vi "ThresholdArray.vi"(9 "Threshold":dbl, 11 "Input Array":dbl[](array[numeric])) -> (3 "Thresholded Array":dbl[](array[numeric]))   [LabVIEW 2014]
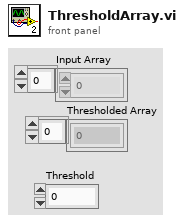
[diagram p1: front panel]
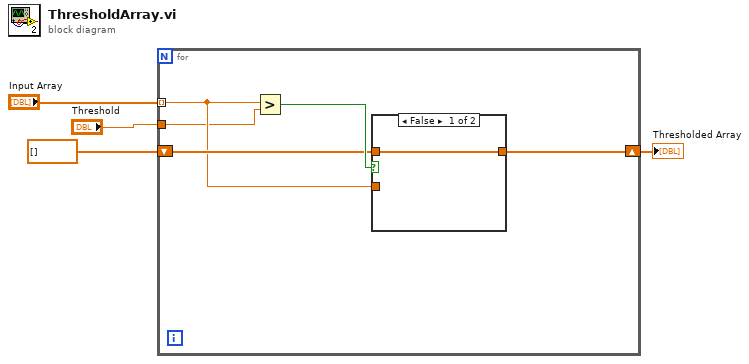
[diagram p0: block diagram]
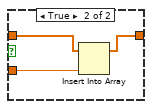
[diagram p2: hidden frame]
diagram:
  n1 = for {
    tunnel: "Input Array" -> [w7] mode=indexing
    shift-right: [w6] -> w2
    shift-left: dbl[] [] -> [w8]
    tunnel: "Threshold" -> [w5]
    n2 = Greater?(x=w7, y=w5) -> (0:w9:bool)
    n3 = case shown="False" w9 {
      tunnel: w8 -> [w10 w13]
      tunnel: w7 -> [_ w12]
      tunnel: [w10 w11] -> w6
      frame False {
      }
      frame True {
        n4 = Insert Into Array(array=w13, new element=w12) -> (w11:dbl[])  [unwired: 1 in]
      }
    }
  }
  "Thresholded Array" <- w2
